vi "Export Project-Screen.vi"(8 "error in (no error)":errorcluster, 9 "File Prefix":string="Proj1_MOD", 10 "Destination Folder":path=path "C:/Users/Public/Documents/National Instruments/NI VeriStand 2013/Projects/Multi_WS", 11 "File Path - Source":path=path "C:/Users/Public/Documents/National Instruments/NI VeriStand 2013/Projects/Multi_WS/Proj1.nivsproj") -> (0 "error out":errorcluster)   [LabVIEW 2014]
uses:
  _typedefs/_saveasProj_States.ctl
  <vilib>/xml/Load XML File.vi
  <vilib>/xml/Close Reference(Node).vi
  <vilib>/xml/NI_XML.lvlib
  <resource>/objmgr/DOMUserDefRef.rc
panel:
  out "Node Value":string
  out "parse errors":string
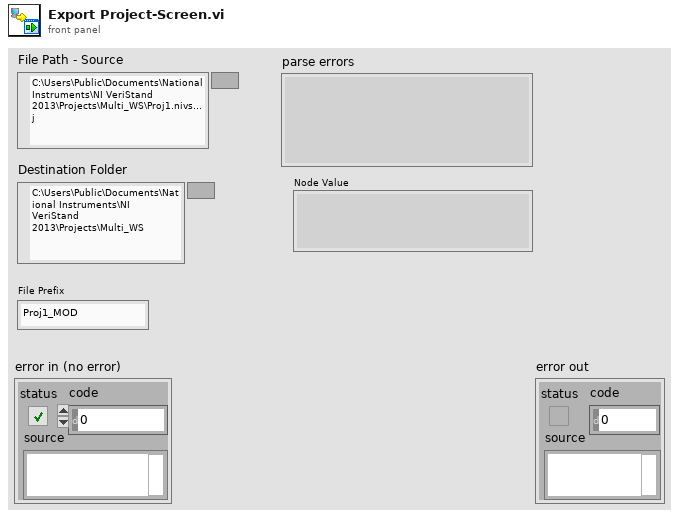
[diagram p1: front panel]
types:
  T1 = typedef "_saveasProj_States.ctl" = enum16{"Initialize", "Replace Workspace Info", "Replace Dependencies", "Save Changes", "Cleanup"}
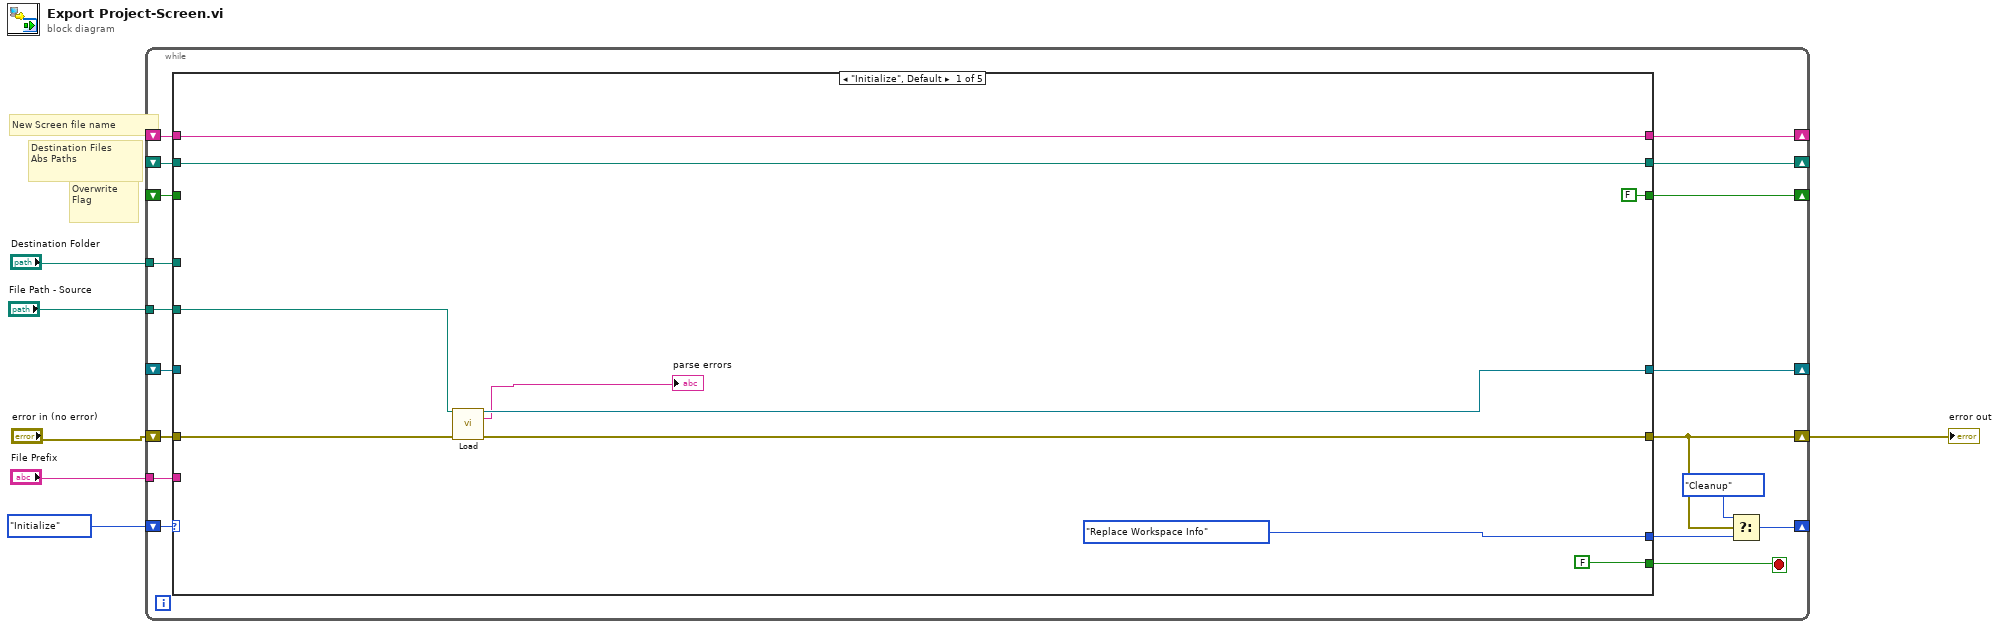
[diagram p0: block diagram]
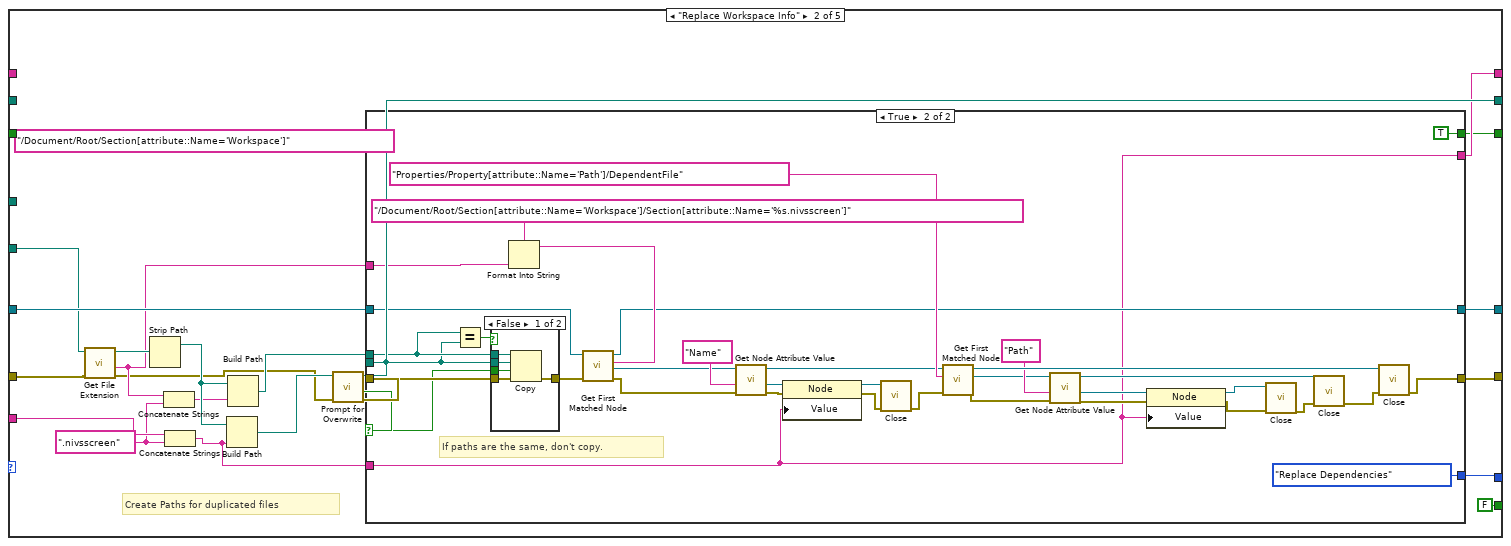
[diagram p2: hidden frame]
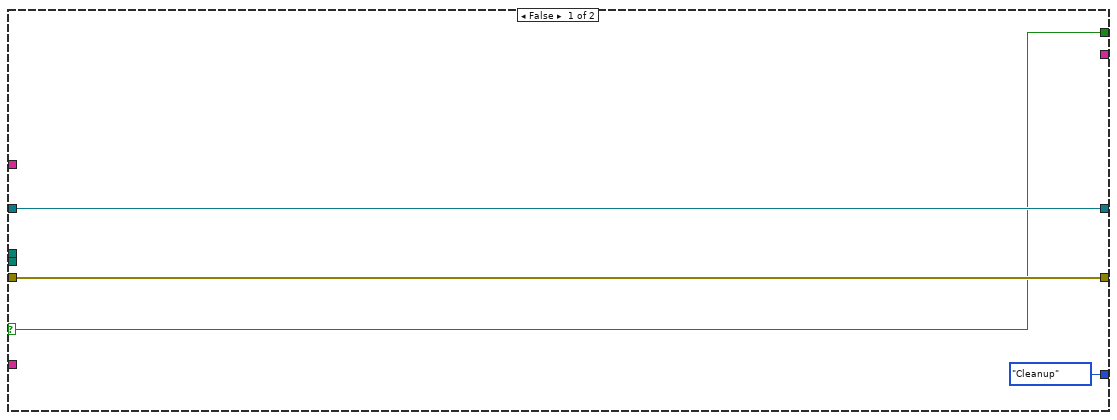
[diagram p3: hidden frame]
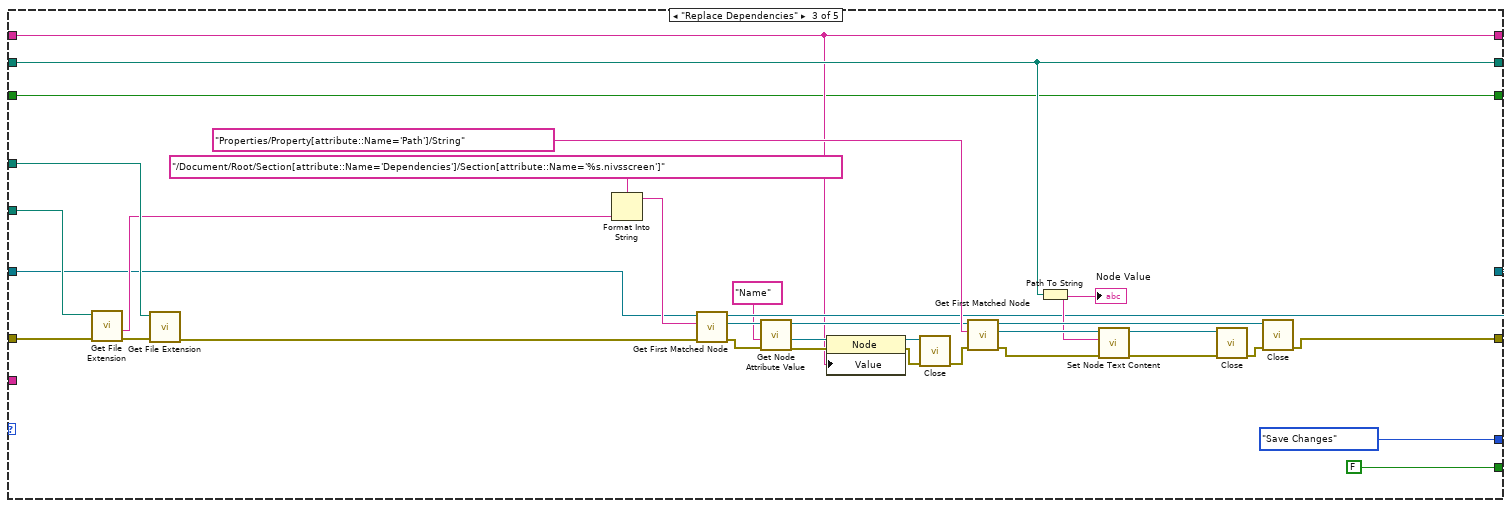
[diagram p5: hidden frame]
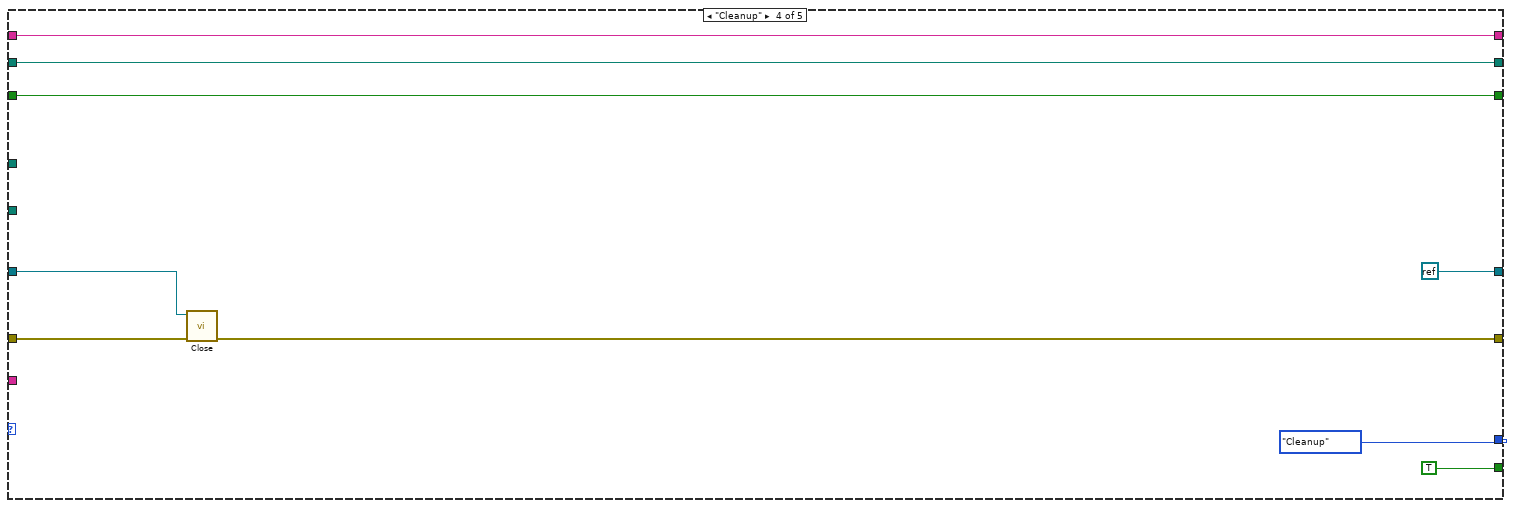
[diagram p6: hidden frame]
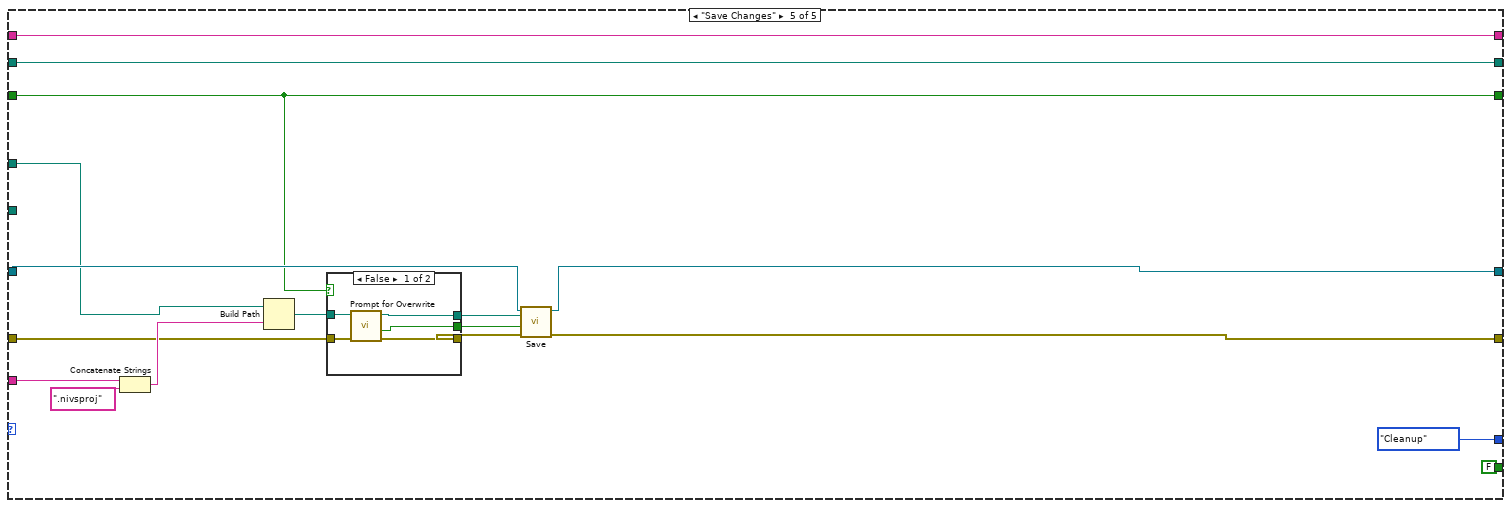
[diagram p7: hidden frame]
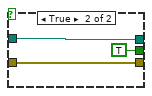
[diagram p8: hidden frame]
diagram:
  # "Overwrite\nFlag"
  # "New Screen file name"
  # "Destination Files\nAbs Paths"
  n1 = while {
    shift-right: [w22] -> _
    shift-left: _saveasProj_States."Initialize" -> [w24]
    tunnel: "File Path - Source" -> [w21]
    shift-right: [w20] -> _
    shift-left: _ -> [w18]
    shift-right: [w7] -> w1
    shift-left: "error in (no error)" -> [w19]
    tunnel: "Destination Folder" -> [w16]
    tunnel: "File Prefix" -> [w15]
    shift-right: [w14] -> _
    shift-left: _ -> [w13]
    shift-right: [w11] -> _
    shift-left: _ -> [w10]
    shift-right: [w9] -> _
    shift-left: _ -> [w8]
    stop <- w17 stop-if-true
    n2 = case shown="\"Initialize\", Default" w24 {
      tunnel: w21 -> [w34 w52 w131 _ _]
      tunnel: [w33 w53 w115 refnum<k0> refnum w160] -> w20
      tunnel: [w32 w51 w114 w138 w159] -> w7
      tunnel: w19 -> [w27 w54 w132 w144 w150]
      tunnel: w18 -> [_ w55 w117 w143 w161]
      tunnel: [_saveasProj_States."Replace Workspace Info" ("f") w56 _saveasProj_States."Save Changes" ("f") _saveasProj_States."Cleanup" ("f") _saveasProj_States."Cleanup" ("f")] -> w12
      tunnel: [FALSE FALSE FALSE TRUE FALSE] -> w17
      tunnel: w16 -> [_ _ w130 _ w153]
      tunnel: w15 -> [_ w49 _ _ w155]
      tunnel: [w28 w39 w118 w139 w152] -> w14
      tunnel: w13 -> [w28 _ w118 w139 w152]
      tunnel: [w26 w36 w104 w137 w147] -> w11
      tunnel: w10 -> [w26 _ w104 w137 w147]
      tunnel: [FALSE w35 w103 w136 w146] -> w9
      tunnel: w8 -> [_ _ w103 w136 w146]
      frame "Initialize", Default {
        n3 = call-poly <vilib>:"Load.vi"("path to XML document"=w34, "error in (no error)"=w27) -> ("DOM document out"=w33:refnum<k20>, "parse errors"=→"parse errors":string, "error out"=w32:errorcluster)  [unwired: 11 in]
      }
      frame "Replace Workspace Info" {
        (unwired) "/Document/Root/Section[attribute::Name='Workspace']" ("XPath expression")
        w47 = ".nivsscreen" ("string")
        # "Create Paths for duplicated files"
        n4 = call <vilib>:"Get File Extension.vi"("error in (no error)"=w54, "file"=w52) -> ("error out"=w41:errorcluster, "filename without extension"=w48:string, "dup file"=w50:path)  [unwired: 6 in, 1 out]
        n5 = Strip Path(path=w50) -> (stripped path=w46:path)  [unwired: 1 out]
        n6 = Concatenate Strings(w48, w47) -> (w45:string)
        n7 = Concatenate Strings(w49, w47) -> (w43:string)
        n8 = Build Path(base path=w46, name or relative path=w43) -> (appended path=w42:path)
        n9 = Build Path(base path=w46, name or relative path=w45) -> (appended path=w44:path)
        n10 = call "Prompt for Overwrite.vi"("error in (no error)"=w41, "path"=w42) -> ("error out"=w40:errorcluster, "Overwrite"=w37:bool, "dup path"=w39:path)  [unwired: 6 in, 1 out]
        n11 = case shown="True" w37 {
          selector: w37 -> [w57 w73]
          tunnel: [_saveasProj_States."Cleanup" ("f") _saveasProj_States."Replace Dependencies" ("f")] -> w56
          tunnel: w55 -> [w59 w70]
          tunnel: [w59 w72] -> w53
          tunnel: [w58 w69] -> w51
          tunnel: w48 -> [_ w75]
          tunnel: w44 -> [_ w63]
          tunnel: w43 -> [_ w65]
          tunnel: w40 -> [w58 w74]
          tunnel: w39 -> [_ w62]
          tunnel: [_ w65] -> w36
          tunnel: [w57 TRUE] -> w35
          frame False {
          }
          frame True {
            # "If paths are the same, don't copy."
            n12 = Equal?(x=w63, y=w62) -> (x = y?=w61:bool)
            n13 = case shown="False" w61 {
              tunnel: w74 -> [w101 w102]
              tunnel: w73 -> [w100 _]
              tunnel: [w99 w102] -> w71
              tunnel: w63 -> [w98 _]
              tunnel: w62 -> [w97 _]
              frame False {
                n14 = Copy(8:w101, 9:w100, 10:w97, 11:w98) -> (0:w99:errorcluster)  [unwired: 1 in, 2 out]
              }
              frame True {
              }
            }
            n15 = Format Into String(format string="/Document/Root/Section[attribute::Name='Workspace']/Section[attribute::Name='%s.nivsscreen']", w75) -> (resulting string=w94:string)  [unwired: 2 in, 1 out]
            n16 = call <vilib>:"Get First Matched Node.vi"("error in (no error)"=w71, "XPath expression"=w94, "node in"=w70) -> ("error out"=w92:errorcluster, "node result"=w81:refnum<k20>, "node out"=w72:refnum<k20>)  [unwired: 6 in]
            n17 = call "Get Node Attribute Value.vi"("error in (no error)"=w92, "Attribute Name"="Name", "Node In"=w81) -> ("error out"=w89:errorcluster, "Attribute Refnum"=w90:refnum<k20>, "Node Out"=w88:refnum<k20>)  [unwired: 6 in]
            n18 = property class="Node"(reference=w90, error in=w89, "Value"=w65) -> (reference out=w87:refnum<k20>, error out=w86:errorcluster)
            n19 = call-poly <vilib>:"Close.vi"("error in (no error)"=w86, "node"=w87) -> ("error out"=w85:errorcluster)  [unwired: 7 in]
            n20 = call <vilib>:"Get First Matched Node.vi"("error in (no error)"=w85, "XPath expression"="Properties/Property[attribute::Name='Path']/DependentFile" ("format string"), "node in"=w88) -> ("error out"=w67:errorcluster, "node result"=w68:refnum<k20>, "node out"=w82:refnum<k20>)  [unwired: 6 in]
            n21 = call "Get Node Attribute Value.vi"("error in (no error)"=w67, "Attribute Name"="Path", "Node In"=w68) -> ("error out"=w78:errorcluster, "Attribute Refnum"=w79:refnum<k20>, "Node Out"=w76:refnum<k20>)  [unwired: 6 in]
            n22 = property class="Node"(reference=w79, error in=w78, "Value"=w65) -> (reference out=w83:refnum<k20>, error out=w84:errorcluster)
            n23 = call-poly <vilib>:"Close.vi"("error in (no error)"=w84, "node"=w83) -> ("error out"=w77:errorcluster)  [unwired: 7 in]
            n24 = call-poly <vilib>:"Close.vi"("error in (no error)"=w77, "node"=w76) -> ("error out"=w66:errorcluster)  [unwired: 7 in]
            n25 = call-poly <vilib>:"Close.vi"("error in (no error)"=w66, "node"=w82) -> ("error out"=w69:errorcluster)  [unwired: 7 in]
          }
        }
      }
      frame "Replace Dependencies" {
        n26 = call <vilib>:"Get File Extension.vi"("error in (no error)"=w132, "file"=w131) -> ("error out"=w133:errorcluster, "filename without extension"=w128:string)  [unwired: 6 in, 2 out]
        n27 = call <vilib>:"Get File Extension.vi"("error in (no error)"=w133, "file"=w130) -> ("error out"=w116:errorcluster)  [unwired: 6 in, 3 out]
        n28 = Format Into String(format string="/Document/Root/Section[attribute::Name='Dependencies']/Section[attribute::Name='%s.nivsscreen']" ("XPath expression"), w128) -> (resulting string=w127:string)  [unwired: 2 in, 1 out]
        n29 = call <vilib>:"Get First Matched Node.vi"("error in (no error)"=w116, "XPath expression"=w127, "node in"=w117) -> ("error out"=w112:errorcluster, "node result"=w113:refnum<k20>, "node out"=w115:refnum<k20>)  [unwired: 6 in]
        n30 = call "Get Node Attribute Value.vi"("error in (no error)"=w112, "Attribute Name"="Name", "Node In"=w113) -> ("error out"=w109:errorcluster, "Attribute Refnum"=w111:refnum<k20>, "Node Out"=w110:refnum<k20>)  [unwired: 6 in]
        n31 = property class="Node"(reference=w111, error in=w109, "Value"=w104) -> (reference out=w106:refnum<k20>, error out=w107:errorcluster)
        n32 = call-poly <vilib>:"Close.vi"("error in (no error)"=w107, "node"=w106) -> ("error out"=w105:errorcluster)  [unwired: 7 in]
        n33 = call <vilib>:"Get First Matched Node.vi"("error in (no error)"=w105, "XPath expression"="Properties/Property[attribute::Name='Path']/String", "node in"=w110) -> ("error out"=w122:errorcluster, "node result"=w123:refnum<k20>, "node out"=w124:refnum<k20>)  [unwired: 6 in]
        n34 = Path To String(path=w118) -> (string=w119:string)
        "Node Value" <- w119
        n35 = call "Set Node Text Content.vi"("error in (no error)"=w122, "node text"=w119, "node in"=w123) -> ("error out"=w120:errorcluster, "node out"=w121:refnum<k20>)  [unwired: 7 in]
        n36 = call-poly <vilib>:"Close.vi"("error in (no error)"=w120, "node"=w121) -> ("error out"=w125:errorcluster)  [unwired: 7 in]
        n37 = call-poly <vilib>:"Close.vi"("error in (no error)"=w125, "node"=w124) -> ("error out"=w114:errorcluster)  [unwired: 7 in]
      }
      frame "Cleanup" {
        n38 = call-poly <vilib>:"Close.vi"("error in (no error)"=w144, "node"=w143) -> ("error out"=w138:errorcluster)  [unwired: 7 in]
      }
      frame "Save Changes" {
        n39 = Concatenate Strings(w155, ".nivsproj" ("string")) -> (w156:string)
        n40 = Build Path(base path=w153, name or relative path=w156) -> (appended path=w151:path)
        n41 = case shown="False" w146 {
          tunnel: w151 -> [w166 w169]
          tunnel: w150 -> [w165 w168]
          tunnel: [w164 w168] -> w149
          tunnel: [w163 w169] -> w148
          tunnel: [w162 TRUE ("Overwrite")] -> w145
          frame False {
            n42 = call "Prompt for Overwrite.vi"("error in (no error)"=w165, "path"=w166) -> ("error out"=w164:errorcluster, "Overwrite"=w162:bool, "dup path"=w163:path)  [unwired: 6 in, 1 out]
          }
          frame True {
          }
        }
        n43 = call <vilib>:"Save.vi"("error in (no error)"=w149, "overwrite file (True)"=w145, "XML file path"=w148, "DOM document in"=w161) -> ("error out"=w159:errorcluster, "DOM document out"=w160:refnum<k20>)  [unwired: 5 in, 1 out]
      }
    }
    n44 = Select(t=_saveasProj_States."Cleanup", s=w7, f=w12) -> (s? t:f=w22:T1)
  }
  "error out" <- w1
